vi "Obtain Broadcast Events.vi"(8 "error in":errorcluster, 10 "Create New? (F)":bool) -> (0 "error out":errorcluster, 2 "Settings Editor Broadcast Events":T1)   [LabVIEW 2020, in "Settings Editor.lvlib"]
doc: "This VI Obtains/Creates the Broadcast events that will be used for other modules to register to receive messages from the module that owns this VI.\n\n<b>NOTE</b>: The contents of this VI are automatically generated and modified by the <b>Tools > DQMH Consortium > DQMH</b> utilities. Consider using those utilities instead of making your own modifications to this VI.\n_____\nBased on DQMH Project Template 4.0.0.47.\n_____\nBased on DQMH Project Template 7.0.1.1316."
uses:
  Settings Editor.lvlib
  Broadcast Events--cluster.ctl
  Did Init Argument--cluster.ctl
  Status Updated Argument--cluster.ctl
  Error Reported Argument--cluster.ctl
  Stop Argument--cluster.ctl
  Get Module Execution Status Argument--cluster.ctl
  Update Application Settings (Reply Payload)--cluster.ctl
  Settings--cluster.ctl
  CML Shared/Signal Type--enum.ctl
  CML Shared/Calibration Values--cluster.ctl
  CML Shared/CML Shared.lvlib
panel:
  # "NOTE: The contents of this VI are automatically generated and modified by the Tools > DQMH Consortium > DQMH utilities. Consider using those utilities instead of making your own modifications to this VI."
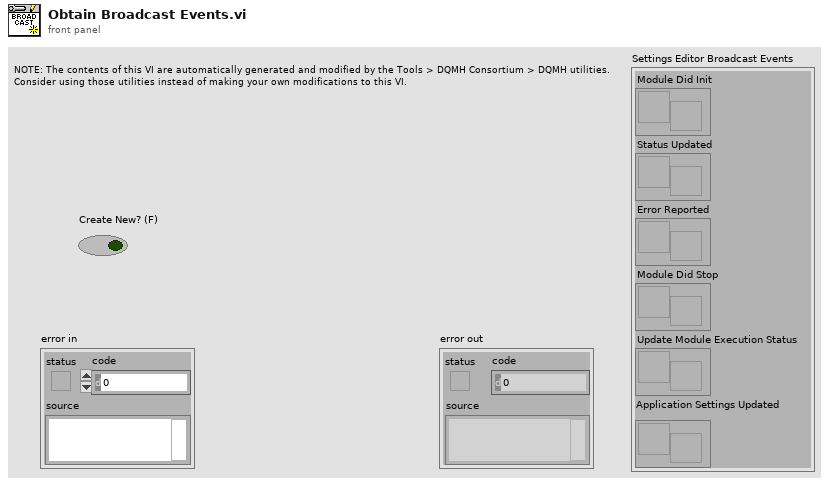
[diagram p1: front panel]
types:
  T1 = typedef "Settings Editor.lvlib/Broadcast Events--cluster.ctl" = cluster{"Module Did Init":refnum<user-event>, "Status Updated":refnum<user-event>, "Error Reported":refnum<user-event>, "Module Did Stop":refnum<user-event>, "Update Module Execution Status":refnum<user-event>, "Application Settings Updated":refnum<user-event>}
  T2 = typedef "Settings Editor.lvlib/Update Application Settings (Reply Payload)--cluster.ctl" = cluster{"Settings":T3, "error":errorcluster}
  T3 = typedef "Settings Editor.lvlib/Settings--cluster.ctl" = cluster{"Signal Type":T4, "Calibration Array":T5[], "Log File Base Path":path}
  T4 = typedef "CML Shared.lvlib/Signal Type--enum.ctl" = enum16{"Sine Wave", "Square with Noise"}
  T5 = typedef "CML Shared.lvlib/Calibration Values--cluster.ctl" = cluster{"Slope":dbl, "Offset":dbl}
  T6 = typedef "Settings Editor.lvlib/Get Module Execution Status Argument--cluster.ctl" = cluster{"Running?":bool}
  T7 = typedef "Settings Editor.lvlib/Stop Argument--cluster.ctl" = cluster{"Origin":string, "Exit via Stop Module Req?":bool, "Wait for Module to stop?":bool}
  T8 = typedef "Settings Editor.lvlib/Error Reported Argument--cluster.ctl" = cluster{"Error":errorcluster, "Additional Information":string, "Module Name":string}
  T9 = typedef "Settings Editor.lvlib/Status Updated Argument--cluster.ctl" = cluster{"Status":string}
  T10 = typedef "Settings Editor.lvlib/Did Init Argument--cluster.ctl" = cluster{"Init?":bool, "Info":string}
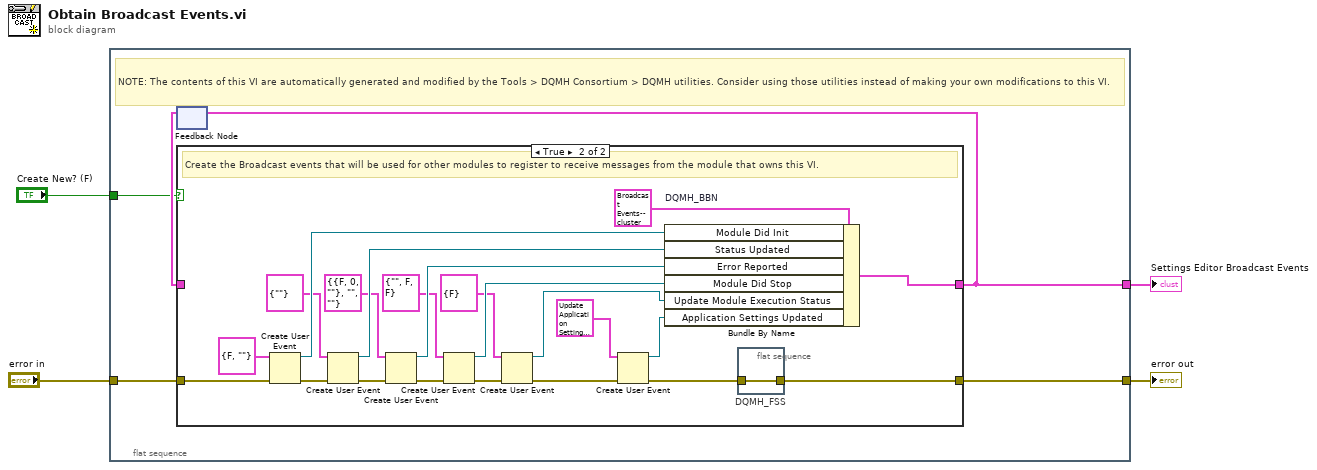
[diagram p0: block diagram]
diagram:
  n1 = flat-sequence {
    tunnel: [w9] -> w4
    tunnel: "error in" -> [w8]
    tunnel: [w6] -> w2
    tunnel: "Create New? (F)" -> [w5]
    frame #0 {
      # "NOTE: The contents of this VI are automatically generated and modified by the Tools > DQMH Consortium > DQMH utilities. Consider using those utilities instead of making your own modifications to this VI."
      n2 = feedback #1() -> (w7:T1)  [unwired: 1 in]
      n3 = case shown="True" w5 {
        tunnel: [w10 w18] -> w9
        tunnel: w8 -> [w10 w33]
        tunnel: [w11 w30] -> w6
        tunnel: w7 -> [w11 _]
        frame False {
          # "Obtain the Broadcast events that were created in a previous call to this VI."
        }
        frame True {
          # "Create the Broadcast events that will be used for other modules to register to receive messages from the module that owns this VI."
          n4 = Create User Event(user event datatype=T10 {"Init?"=FALSE, "Info"=""} ("Did Init Argument"), error in=w33) -> (user event=w31:refnum<user-event>, error out=w28:errorcluster)
          n5 = Create User Event(user event datatype=T9 {"Status"=""} ("Status Updated Argument"), error in=w28) -> (user event=w25:refnum<user-event>, error out=w27:errorcluster)
          n6 = Create User Event(user event datatype=T8 {"Error"={"status"=FALSE, "code"=0, "source"=""}, "Additional Information"="", "Module Name"=""} ("Error Reported Argument"), error in=w27) -> (user event=w22:refnum<user-event>, error out=w24:errorcluster)
          n7 = Create User Event(user event datatype=T7 {"Origin"="", "Exit via Stop Module Req?"=FALSE, "Wait for Module to stop?"=FALSE} ("Stop Argument"), error in=w24) -> (user event=w20:refnum<user-event>, error out=w19:errorcluster)
          n8 = Create User Event(user event datatype=T6 {"Running?"=FALSE} ("Get Module Execution Status Argument"), error in=w19) -> (user event=w16:refnum<user-event>, error out=w17:errorcluster)
          n9 = Create User Event(user event datatype=T2 {"Settings"={"Signal Type"=enum."Sine Wave", "Calibration Array"=[], "Log File Base Path"=path ""}, "error"={"status"=FALSE, "code"=0, "source"=""}} ("Update Application Settings (Reply Payload)"), error in=w17) -> (user event=w13:refnum<user-event>, error out=w14:errorcluster)
          n10 = Bundle By Name "DQMH_BBN"(cluster=T1 {"Module Did Init"=refnum, "Status Updated"=refnum, "Error Reported"=refnum, "Module Did Stop"=refnum, "Update Module Execution Status"=refnum, "Application Settings Updated"=refnum} ("output cluster"), "Module Did Init"=w31, "Status Updated"=w25, "Error Reported"=w22, "Module Did Stop"=w20, "Update Module Execution Status"=w16, "Application Settings Updated"=w13) -> (w30:T1)
          n11 = flat-sequence "DQMH_FSS" {
            tunnel: w14 -> [w34]
            tunnel: [w34] -> w18
            frame #0 {
            }
          }
        }
      }
      n12 = feedback-in #1(w6) -> ()
    }
  }
  "Settings Editor Broadcast Events" <- w2
  "error out" <- w4
